vi "GFITS_WriteImNameToFile.vi"(6 "max bytes size":i32=200000, 7 "id":string, 8 "error in (no error)":errorcluster, 9 "Status":string, 10 "Image":string, 11 "Path":path) -> (0 "error out":errorcluster)   [LabVIEW 2016]
uses:
  <vilib>/Utility/config.llb/Write Key (String).vi
  <vilib>/Utility/config.llb/NI_LVConfig.lvlib
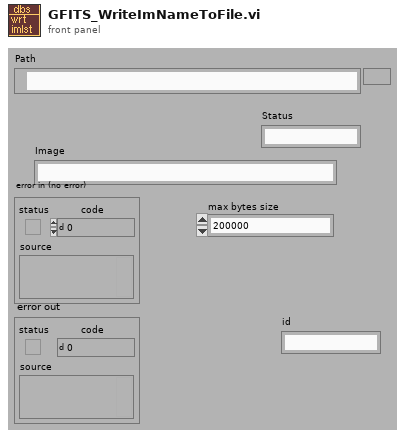
[diagram p1: front panel]
types:
  T1 = typedef "NI_LVConfig.lvlib/Config Data RefNum.ctl" = refnum<k1>
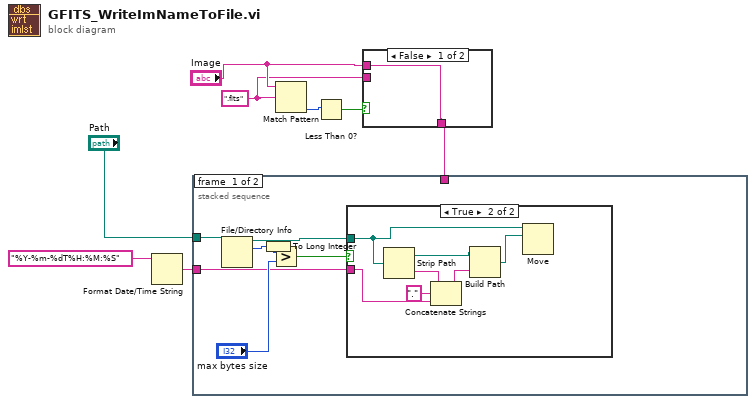
[diagram p0: block diagram]
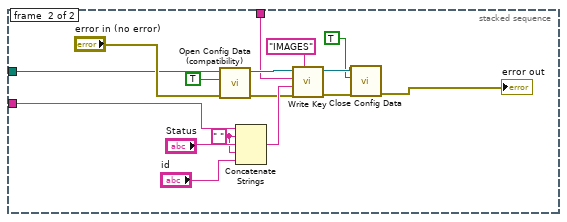
[diagram p3: hidden frame]
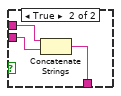
[diagram p4: hidden frame]
diagram:
  w5 = ".fits" ("regular expression")
  n1 = Format Date/Time String(time format string (%c)="%Y-%m-%dT%H:%M:%S") -> (date/time string=w1:string)  [unwired: 2 out]
  n2 = Match Pattern(string="Image", regular expression=w5) -> (offset past match=w8:i32)  [unwired: 4 out]
  n3 = Less Than 0?(x=w8) -> (x < 0?=w7:bool)
  n4 = case shown="False" w7 {
    tunnel: "Image" -> [w9 w12]
    tunnel: w5 -> [_ w11]
    tunnel: [w9 w10] -> w4
    frame False {
    }
    frame True {
      n5 = Concatenate Strings(w12, w11) -> (w10:string)
    }
  }
  n6 = stacked-sequence {
    tunnel: w4 -> [_ w31]
    tunnel: "Path" -> [w17 w30]
    tunnel: w1 -> [w14 w29]
    frame #0 {
      n7 = File/Directory Info(path=w17) -> (path out=w15:path, size=w13:i64)  [unwired: 1 in, 5 out]
      n8 = To Long Integer(number=w13) -> (32bit integer=w18:i32)
      n9 = Greater?(x=w18, y="max bytes size") -> (0:w16:bool)
      n10 = case shown="True" w16 {
        tunnel: w15 -> [_ w26]
        tunnel: w14 -> [_ w24]
        frame False {
        }
        frame True {
          n11 = Strip Path(path=w26) -> (stripped path=w21:path, name=w25:string)
          n12 = Concatenate Strings(w25, "." ("string"), w24) -> (w20:string)
          n13 = Build Path(base path=w21, name or relative path=w20) -> (appended path=w22:path)
          n14 = Move(source path=w26, 10:w22) -> ()  [unwired: 1 in, 5 out]
        }
      }
    }
    frame #1 {
      w28 = " " ("string")
      n15 = call <vilib>:"Open Config Data (compatibility).vi"("error in (no error)"="error in (no error)", "create file if necessary (T)"=TRUE ("create file if necessary? (T)"), "configuration file path"=w30) -> ("error out"=w36:errorcluster, "refnum"=w42:T1)  [unwired: 6 in, 1 out]
      n16 = Concatenate Strings(w29, w28, "Status", w28, "id") -> (w39:string)
      n17 = call-poly <vilib>:"Write Key.vi"("section"="IMAGES", "error in (no error)"=w36, "value"=w39, "key"=w31, "refnum"=w42) -> ("error out"=w37:errorcluster, "refnum out"=w38:T1)  [unwired: 1 in, 4 out]
      n18 = call <vilib>:"Close Config Data.vi"("error in (no error)"=w37, "write file if changed (T)"=TRUE ("write configuration file? (F)"), "refnum"=w38) -> ("error out"=→"error out":errorcluster)  [unwired: 8 out]
    }
  }
